vi "Send Button Pressed.vi"(7 "Message Priority (Normal)":T2=enum."Normal", 8 "error in (no error)":errorcluster, 9 "Data":variant, 10 "Button":T1, 11 "Message Enqueuer":refnum<class "Message Enqueuer.lvclass">) -> (0 "error out":errorcluster, 3 "Message Enqueuer out":refnum<class "Message Enqueuer.lvclass">)   [LabVIEW 2026, in "TALOS.lvlib" / "Guardian.lvlib" / "Button Pressed Msg.lvclass"]
doc: "This VI sends the message to an actor."
uses:
  Button Pressed Msg.lvclass
  builds/Actor Framework PPL/Actor Framework.lvlibp/1abvi3w/vi.lib/ActorFramework/Message Enqueuer/Message Enqueuer.lvclass
  builds/Actor Framework PPL/Actor Framework.lvlibp/1abvi3w/vi.lib/ActorFramework/Message Enqueuer/Message Priority.ctl
  Guardian/Buttons_UI.ctl
  Button Pressed Msg.lvclass/Button Pressed Msg.ctl
  C:/LabVIEW Code/TALOS/builds/Actor Framework PPL/Actor Framework.lvlibp/1abvi3w/vi.lib/ActorFramework/Message/Message.lvclass
  Guardian/Guardian.lvclass
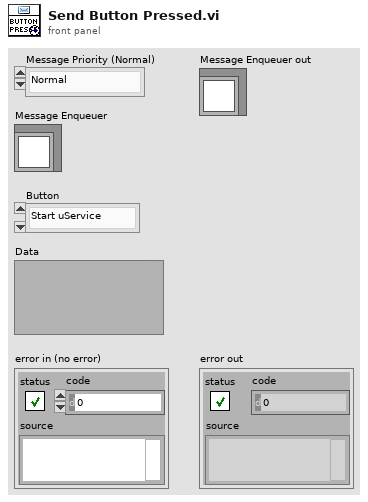
[diagram p1: front panel]
types:
  T1 = typedef "TALOS.lvlib/Guardian.lvlib/Guardian.lvclass/Buttons_UI.ctl" = enum16{"Start uService", "Kill uService", "Stop uService", "Stop", "Start online checks", "Stop online checks", "Send Pat to all GDs", "Reload INI files", "Update from GIT", "RUN", "Reset ABORT", "Check Bearer", "Send I Exist", "Change Run Config", "Add uSs from Config", "Realign uSs from Config", "Send Run Config to GD"}
  T2 = typedef "Actor Framework.lvlibp/Message Enqueuer.lvclass/Message Priority.ctl" = enum16{"Low", "Normal", "High"}
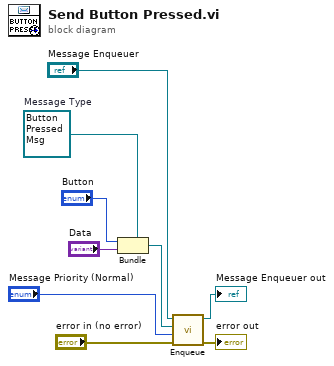
[diagram p0: block diagram]
diagram:
  w6 = refnum<class "Button Pressed Msg.lvclass"> refnum  # Message Type
  n1 = Bundle(cluster=w6, "Button", "Data") -> (w5:refnum<class "Button Pressed Msg.lvclass">)
  n2 = call "Enqueue.vi"("error in (no error)"="error in (no error)", "Message Priority (Normal)"="Message Priority (Normal)", "Message"=w5, "Message Enqueuer in"="Message Enqueuer") -> ("error out"=→"error out":errorcluster, "Message Enqueuer out"=→"Message Enqueuer out":refnum<class "Message Enqueuer.lvclass">)  [unwired: 6 in]
